vi "VAI Init ADC.vi"(7 "Period":u16, 9 "Channel":u8, 10 "DevIndex":i32, 11 "DevType":i32) -> (3 "function return":i32)   [LabVIEW 2010, in "ControlADC.lvlib"]
doc: "int WINAPI VAI_InitADC(int DevType, int DevIndex, unsigned char Channel, unsigned short Period);"
uses:
  ControlADC.lvlib
  ControlADC/Ginkgo_Driver.dll
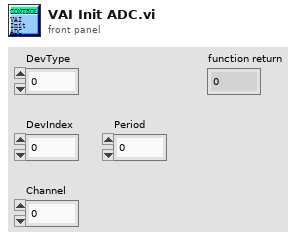
[diagram p1: front panel]
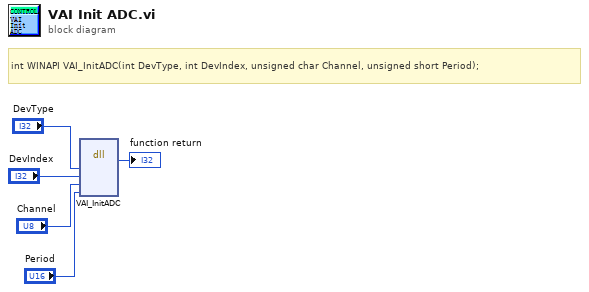
[diagram p0: block diagram]
diagram:
  # "int WINAPI VAI_InitADC(int DevType, int DevIndex, unsigned char Channel, unsigned short Period);"
  n1 = dll-call lib="E:/Project/vt_ginkgo/truck/Ginkgo Driver/vs2010/Ginkgo_USB-I2C&SPI&CAN_API_v2.0.3.3/lib/labview_32bit/ControlADC/Ginkgo_Driver.*" fn="VAI_InitADC"("DevType"="DevType", "DevIndex"="DevIndex", "Channel"="Channel", "Period"="Period") -> (→"function return":i32)  [unwired: 7 in, 2 out]
